vi "Get-storage-buffer-element.vi"(8 "error in (no error)":errorcluster, 10 "Index":i32, 11 "Buffers in":refnum<class "CV-Buffers.lvclass">) -> (0 "error out":errorcluster, 2 "Element ref":T1, 3 "Buffers out":refnum<class "CV-Buffers.lvclass">)   [LabVIEW 2013, in "CameraVision.lvlib" / "CV-Buffers.lvclass"]
uses:
  CV-Buffers.lvclass
  Storage-buffer-refs.ctl
  <vilib>/vision/Image Controls.llb/IMAQ Image.ctl
  CV-Buffers.lvclass/CV-Buffers.ctl
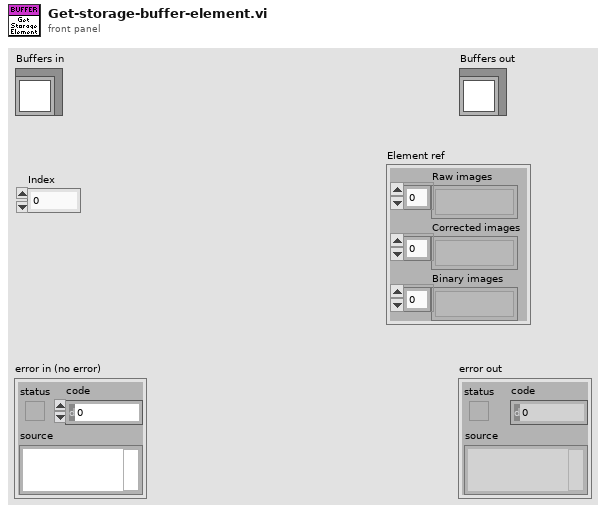
[diagram p1: front panel]
types:
  T1 = typedef "CameraVision.lvlib/CV-Buffers.lvclass/Storage-buffer-refs.ctl" = cluster{"Raw images":T2[], "Corrected images":T2[], "Binary images":T2[]}
  T2 = typedef "IMAQ Image.ctl" = refnum<image>
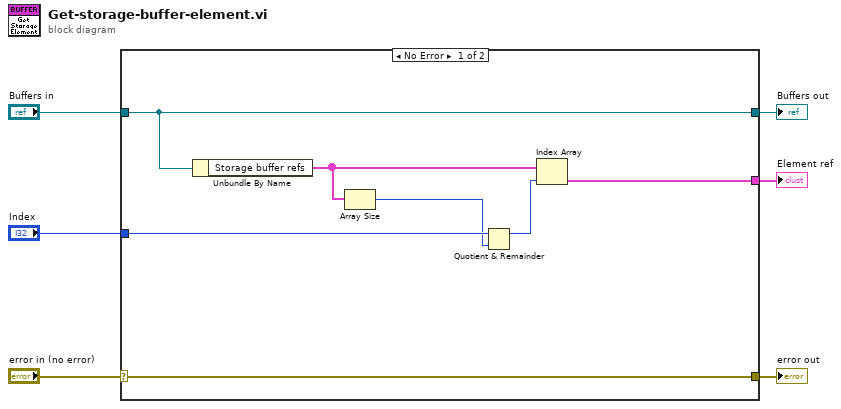
[diagram p0: block diagram]
diagram:
  n1 = case shown="No Error" "error in (no error)" {
    selector: "error in (no error)" -> [w9 w15]
    tunnel: [w9 w15] -> w5
    tunnel: [w13 w14] -> w3
    tunnel: "Buffers in" -> [w13 w14]
    tunnel: "Index" -> [w12 _]
    tunnel: [w8 _] -> w1
    frame No Error {
      n2 = Unbundle By Name(w13) -> ("Storage buffer refs"=w11:T1[])
      n3 = Array Size(array=w11) -> (size(s)=w7:i32)
      n4 = Quotient & Remainder(x=w12, y=w7) -> (x-y*floor(x/y)=w10:i32)  [unwired: 1 out]
      n5 = Index Array(array=w11, index=w10) -> (element=w8:T1)
    }
    frame Error {
    }
  }
  "error out" <- w5
  "Buffers out" <- w3
  "Element ref" <- w1
